vi "Configuration.vi"(11 "Configuration Queue":refnum<queue>) -> ()   [LabVIEW 2013, in "main.lvlib"]
uses:
  main.lvlib
  Controls/Reference AE Control.ctl
  Controls/Reference Cluster.ctl
panel:
  in  "ActivityBox":bool caption="Arbejdstest"
  out "SegmentNumberString":string caption="Nummer"
  out "UndersøgelsesString":string caption="Undersøgelse"
  out "ArmtrykString":string caption="Armtryk"
  in  "Stop":bool
  in  "ListboxLeftSegmentNr":i32(listbox) caption="Venstre"
  in  "ListboxRightSegmentNr":i32(listbox) caption="Højre"
  in  "ListboxMeasurementArea":i32(listbox) caption="Segment"
  in  "ListboxMeasurementTechnique":i32(listbox) caption="Teknik"
  in  "ListboxMeasurementMeth":i32(listbox) caption="Metode"
  in  "TempTwo":dbl caption="#2"
  in  "TempOne":dbl caption="Temperatur"
  in  "PalpationLeft":string(combo)="None" caption="Palpation"
  in  "PalpationRight":string(combo)="None" caption="Palpation"
  in  "LeftArmPressureTable":string[][](table) caption="Venstre"
  in  "RightArmPressureTable":string[][](table) caption="Højre"
  in  "HeightAdjustmentInt":dbl caption="Højdejustering"
  in  "SaveArmPressureBtn":bool caption="Gem"
  in  "Puls":dbl
  # "#1"
  # "#2"
  # "cm"
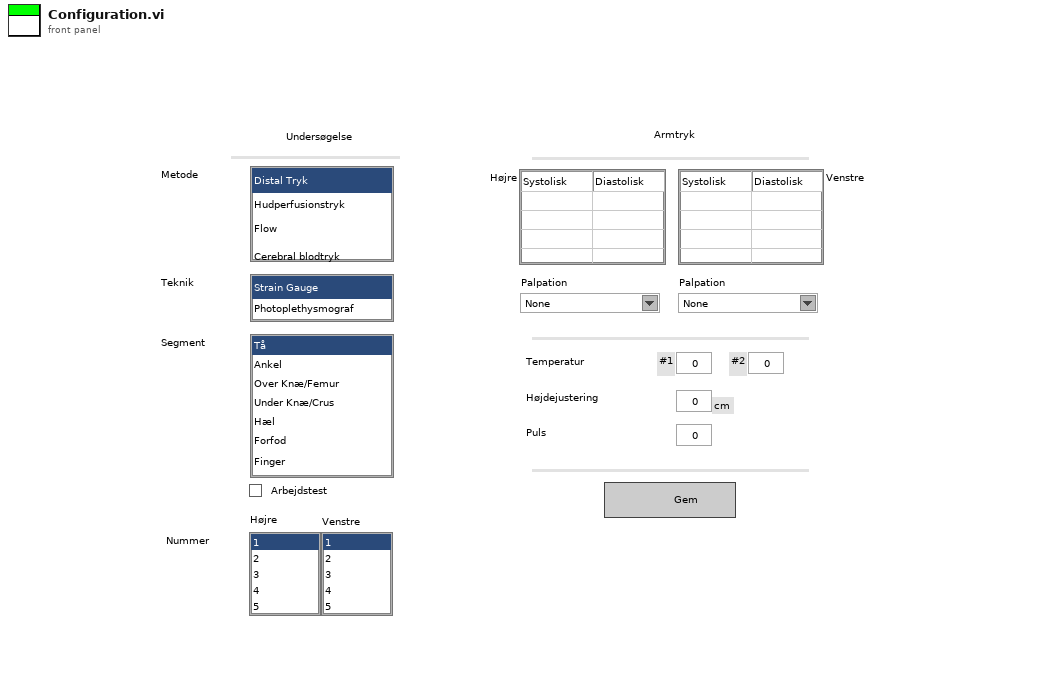
[diagram p1: front panel]
types:
  T1 = typedef "main.lvlib/Reference AE Control.ctl" = enum16{"Initialize", "Set Menu", "Set Profile", "Set Configuration", "Set Configuration_old", "Set Configuration_new", "Set Configuration Method", "Set Acquisition", "Set Data", "Set Journal", "Get"}
  T2 = typedef "main.lvlib/Reference Cluster.ctl" = cluster{"Menu":cluster{"References":cluster{"Stop Acq":refnum<vi>, "MenuExit":refnum<vi>, "MenuStartADC":refnum<vi>, "PersonalInfoString":refnum<vi>, "Profile":refnum<vi>, "Configuration":refnum<vi>, "Acquisition":refnum<vi>, "Data":refnum<vi>, "Journal":refnum<vi>}}, "Profile":cluster{"References":cluster{"Search Patient ID":refnum<vi>, "Name":refnum<vi>, "CommentStr":refnum<vi>, "Listbox Patient ID":refnum<vi>, "ListboxDoctor":refnum<vi>, "ListboxOperator":refnum<vi>, "HospitalName":refnum<vi>, "HospitalDepartment":refnum<vi>, "HospitalAddress":refnum<vi>, "EditHospInfo":refnum<vi>, "Add Patient ID Btn":refnum<vi>, "Query Worklist":refnum<vi>}}, "Configuration":cluster{"References":cluster{"ListboxMeasurementArea":refnum<vi>, "ListboxMeasurementTechnique":refnum<vi>, "ListboxMeasurementMeth":refnum<vi>, "ListboxRightSegmentNr":refnum<vi>, "ListboxLeftSegmentNr":refnum<vi>, "HeightAdjustmentInt":refnum<vi>, "PalpationRight":refnum<vi>, "PalpationLeft":refnum<vi>, "ActivityBox":refnum<vi>}, "New method":cluster{"AddNewMeasurementBtn":refnum<vi>, "Left Time Table":refnum<vi>, "Right Time Table":refnum<vi>}, "Old method":cluster{"LeftArmPressureTable":refnum<vi>, "RightArmPressureTable":refnum<vi>, "SaveArmPressureBtn":refnum<vi>, "Puls":refnum<vi>, "TempTwo":refnum<vi>, "TempOne":refnum<vi>}, "Method":string}, "Acquisition":cluster{"References":cluster{"SegmentAcqString":refnum<vi>, "RingActGraph":refnum<vi>}}, "Data":cluster{"References":cluster{"cmString":refnum<vi>, "AdjustedHeight":refnum<vi>, "Menu":refnum<vi>, "Tangent On/Off":refnum<vi>, "FilterControl":refnum<vi>}}, "Journal":cluster{"References":cluster{"ReportSelection":refnum<vi>, "Data":refnum<vi>, "GenerateReport":refnum<vi>, "Menu":refnum<vi>, "Send To PACS":refnum<vi>}}}
  T3 = cluster{"ListboxMeasurementArea":refnum<vi>, "ListboxMeasurementTechnique":refnum<vi>, "ListboxMeasurementMeth":refnum<vi>, "ListboxRightSegmentNr":refnum<vi>, "ListboxLeftSegmentNr":refnum<vi>, "HeightAdjustmentInt":refnum<vi>, "PalpationRight":refnum<vi>, "PalpationLeft":refnum<vi>, "ActivityBox":refnum<vi>}
  T4 = typedef "LVRectTypeDef.ctl" = cluster{"Left":i16, "Top":i16, "Right":i16, "Bottom":i16}
  T5 = cluster{"sys":dbl, "dia":dbl, "puls":dbl, "date":string, "time":string, "code":string, "serial":string, "temp":dbl, "activity":string}[]
  T6 = cluster{"LeftArmPressureTable":refnum<vi>, "RightArmPressureTable":refnum<vi>, "SaveArmPressureBtn":refnum<vi>, "Puls":refnum<vi>, "TempTwo":refnum<vi>, "TempOne":refnum<vi>}
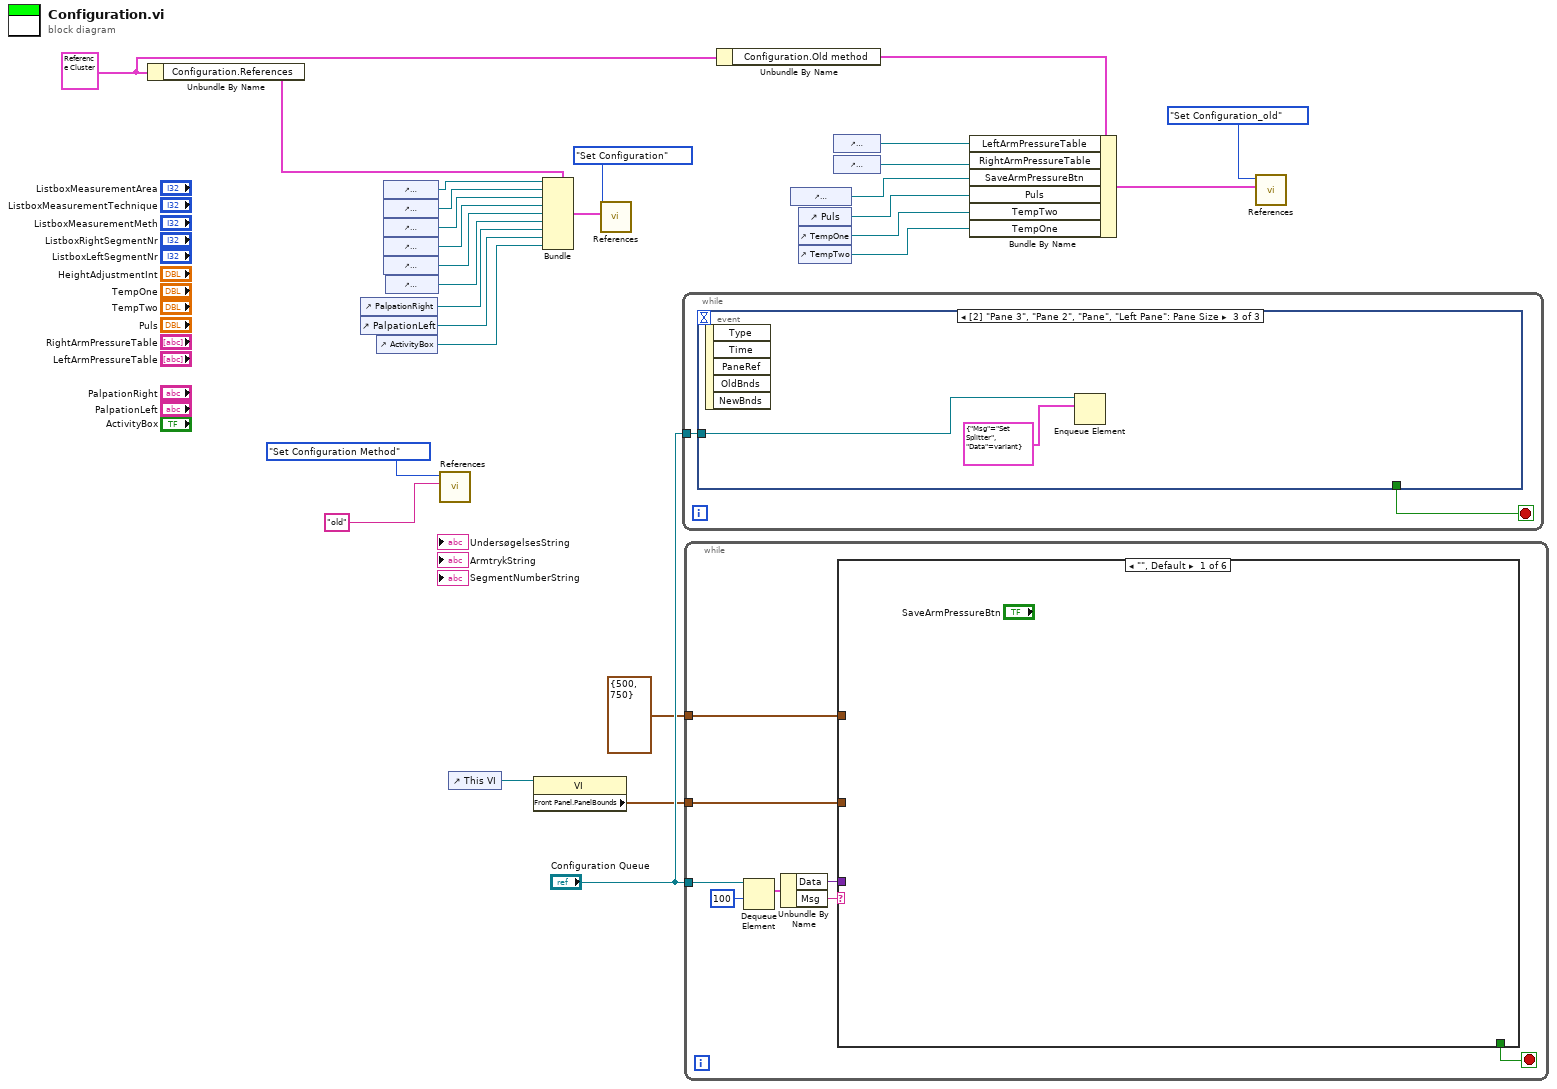
[diagram p0: block diagram]
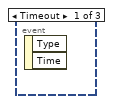
[diagram p2: hidden frame]
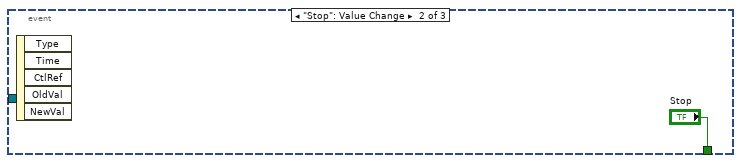
[diagram p3: hidden frame]
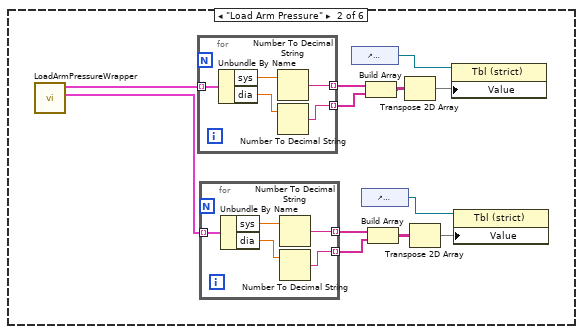
[diagram p4: hidden frame]
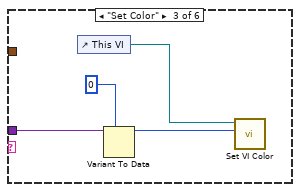
[diagram p5: hidden frame]
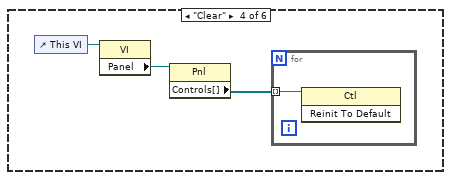
[diagram p6: hidden frame]
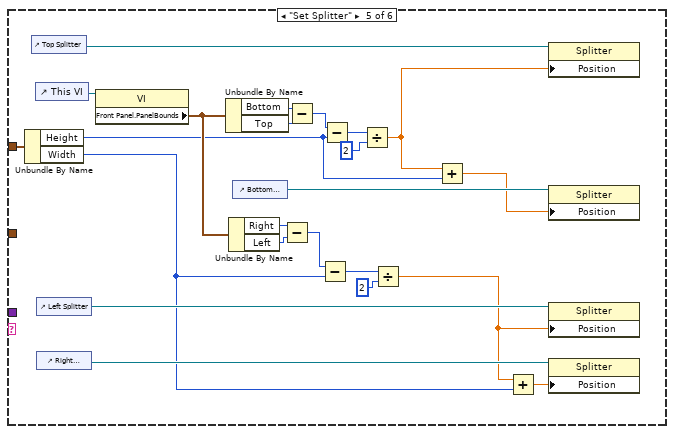
[diagram p7: hidden frame]
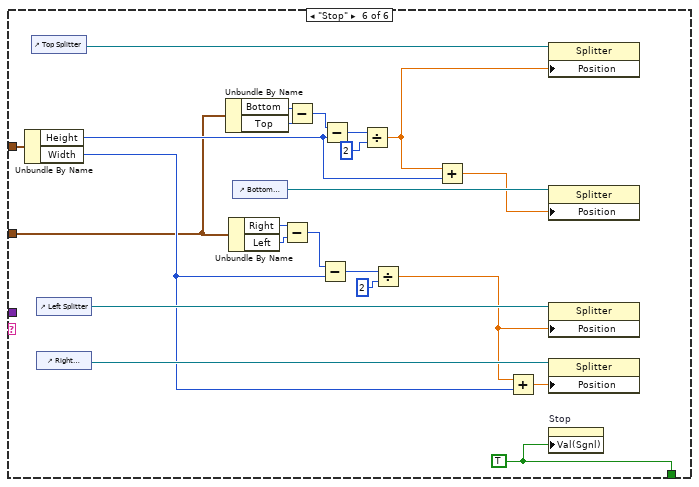
[diagram p8: hidden frame]
diagram:
  w15 = T2 {"Menu"={"References"={"Stop Acq"=refnum, "MenuExit"=refnum, "MenuStartADC"=refnum, "PersonalInfoString"=refnum, "Profile"=refnum, "Configuration"=refnum, "Acquisition"=refnum, "Data"=refnum, "Journal"=refnum}}, "Profile"={"References"={"Search Patient ID"=refnum, "Name"=refnum, "CommentStr"=refnum, "Listbox Patient ID"=refnum, "ListboxDoctor"=refnum, "ListboxOperator"=refnum, "HospitalName"=refnum, "HospitalDepartment"=refnum, "HospitalAddress"=refnum, "EditHospInfo"=refnum, "Add Patient ID Btn"=refnum, "Query Worklist"=refnum}}, "Configuration"={"References"={"ListboxMeasurementArea"=refnum, "ListboxMeasurementTechnique"=refnum, "ListboxMeasurementMeth"=refnum, "ListboxRightSegmentNr"=refnum, "ListboxLeftSegmentNr"=refnum, "HeightAdjustmentInt"=refnum, "PalpationRight"=refnum, "PalpationLeft"=refnum, "ActivityBox"=refnum}, "New method"={"AddNewMeasurementBtn"=refnum, "Left Time Table"=refnum, "Right Time Table"=refnum}, "Old method"={"LeftArmPressureTable"=refnum, "RightArmPressureTable"=refnum, "SaveArmPressureBtn"=refnum, "Puls"=refnum, "TempTwo"=refnum, "TempOne"=refnum}, "Method"=""}, "Acquisition"={"References"={"SegmentAcqString"=refnum, "RingActGraph"=refnum}}, "Data"={"References"={"cmString"=refnum, "AdjustedHeight"=refnum, "Menu"=refnum, "Tangent On/Off"=refnum, "FilterControl"=refnum}}, "Journal"={"References"={"ReportSelection"=refnum, "Data"=refnum, "GenerateReport"=refnum, "Menu"=refnum, "Send To PACS"=refnum}}}
  n1 = Unbundle By Name(w15) -> ("Configuration.References"=w16:T3)
  n2 = control-ref of="PalpationRight"() -> (w5:refnum<vi>)
  n3 = control-ref of="PalpationLeft"() -> (w4:refnum<vi>)
  n4 = control-ref of="ActivityBox"() -> (w3:refnum<vi>)
  n5 = control-ref of="ListboxMeasurementArea"() -> (w28:refnum<vi>)
  n6 = control-ref of="ListboxMeasurementTechnique"() -> (w27:refnum<vi>)
  n7 = control-ref of="ListboxMeasurementMeth"() -> (w26:refnum<vi>)
  n8 = control-ref of="ListboxRightSegmentNr"() -> (w25:refnum<vi>)
  n9 = control-ref of="ListboxLeftSegmentNr"() -> (w24:refnum<vi>)
  n10 = control-ref of="HeightAdjustmentInt"() -> (w23:refnum<vi>)
  n11 = call "References.vi"("variant"="old", "Reference AE Control"=Reference_AE_Control."Set Configuration Method") -> ()  [unwired: 8 in, 2 out]
  n12 = control-ref of="This VI"() -> (w19:refnum<vi>)
  n13 = property class="VI"(reference=w19) -> ("Front Panel.PanelBounds"=w18:T4)  [unwired: 1 in, 2 out]
  n14 = Bundle(cluster=w16, "ListboxMeasurementArea"=w28, "ListboxMeasurementTechnique"=w27, "ListboxMeasurementMeth"=w26, "ListboxRightSegmentNr"=w25, "ListboxLeftSegmentNr"=w24, "HeightAdjustmentInt"=w23, "PalpationRight"=w5, "PalpationLeft"=w4, "ActivityBox"=w3) -> (w21:T3)
  n15 = call "References.vi"("variant"=w21, "Reference AE Control"=Reference_AE_Control."Set Configuration") -> ()  [unwired: 8 in, 2 out]
  n16 = while {
    tunnel: "Configuration Queue" -> [w30]
    stop <- w29 stop-if-true
    n17 = event shown="[2] \"Pane 3\", \"Pane 2\", \"Pane\", \"Left Pane\": Pane Size" {
      selector: _ -> [_ _ _]
      dyn-events: _ -> [_ _ _]
      timeout: _ -> [_ _ _]
      tunnel: w30 -> [_ _ w33]
      tunnel: [_ "Stop" _] -> w29
      event Timeout {
        n18 = event-data() -> ()  [unwired: 1 in, 2 out]
      }
      event "Stop": Value Change {
        n19 = event-data() -> ()  [unwired: 1 in, 5 out]
      }
      event Pane Size {
        n20 = event-data() -> ()  [unwired: 1 in, 5 out]
        n21 = Enqueue Element(queue=w33, element=cluster{"Msg":string, "Data":variant} {"Msg"="Set Splitter", "Data"=variant}) -> ()  [unwired: 2 in, 3 out]
      }
    }
  }
  n22 = while {
    tunnel: "Configuration Queue" -> [w41]
    tunnel: cluster{"Height":i32, "Width":i32} {"Height"=500, "Width"=750} -> [w35]
    tunnel: w18 -> [w34]
    stop <- w38 stop-if-true
    n23 = Dequeue Element(queue=w41, timeout in ms (-1)=100) -> (element=w40:cluster{"Msg":string, "Data":variant})  [unwired: 1 in, 3 out]
    n24 = Unbundle By Name(w40) -> ("Data"=w37:variant, "Msg"=w39:string)
    n25 = case shown="\"\", Default" w39 {
      tunnel: [_ _ _ _ _ w96] -> w38
      tunnel: w37 -> [_ _ w64 _ _ _]
      tunnel: w35 -> [_ _ _ _ w80 w105]
      tunnel: w34 -> [_ _ _ _ _ w95]
      frame "", Default {
      }
      frame "Load Arm Pressure" {
        n26 = call "LoadArmPressureWrapper.vi"() -> ("Armpressure Left"=w48:T5, "Armpressure Right"=w53:T5)  [unwired: 9 in, 1 out]
        n27 = for {
          tunnel: w53 -> [w63] mode=indexing
          tunnel: [w60] -> w52 mode=indexing
          tunnel: [w59] -> w51 mode=indexing
          n28 = Unbundle By Name(w63) -> ("sys"=w62:dbl, "dia"=w61:dbl)
          n29 = Number To Decimal String(number=w62) -> (decimal integer string=w60:string)  [unwired: 1 in]
          n30 = Number To Decimal String(number=w61) -> (decimal integer string=w59:string)  [unwired: 1 in]
        }
        n31 = for {
          tunnel: w48 -> [w58] mode=indexing
          tunnel: [w55] -> w49 mode=indexing
          tunnel: [w54] -> w47 mode=indexing
          n32 = Unbundle By Name(w58) -> ("sys"=w57:dbl, "dia"=w56:dbl)
          n33 = Number To Decimal String(number=w57) -> (decimal integer string=w55:string)  [unwired: 1 in]
          n34 = Number To Decimal String(number=w56) -> (decimal integer string=w54:string)  [unwired: 1 in]
        }
        n35 = control-ref of="RightArmPressureTable"() -> (w50:refnum<vi>)
        n36 = control-ref of="LeftArmPressureTable"() -> (w46:refnum<vi>)
        n37 = Build Array(w52, w51) -> (w45:string[][])
        n38 = Build Array(w49, w47) -> (w43:string[][])
        n39 = Transpose 2D Array(2D array=w45) -> (transposed array=w44:string[][])
        n40 = Transpose 2D Array(2D array=w43) -> (transposed array=w42:string[][])
        n41 = property class="Tbl (strict)"(reference=w50, "Value"=w44) -> ()  [unwired: 1 in, 2 out]
        n42 = property class="Tbl (strict)"(reference=w46, "Value"=w42) -> ()  [unwired: 1 in, 2 out]
      }
      frame "Set Color" {
        n43 = control-ref of="This VI"() -> (w67:refnum<vi>)
        n44 = Variant To Data(type=u32 0 ("Pane Color"), Variant=w64) -> (data=w65:u32)  [unwired: 1 in, 1 out]
        n45 = call "Set VI Color.vi"("Pane Color"=w65, "VI in"=w67) -> ()  [unwired: 10 in]
      }
      frame "Clear" {
        n46 = control-ref of="This VI"() -> (w70:refnum<vi>)
        n47 = property class="VI"(reference=w70) -> ("Panel"=w69:refnum<vi>)  [unwired: 1 in, 2 out]
        n48 = property class="Pnl"(reference=w69) -> ("Controls[]"=w68:refnum<vi>[])  [unwired: 1 in, 2 out]
        n49 = for {
          tunnel: w68 -> [w71] mode=indexing
          n50 = invoke class="Ctl" method="Reinit To Default"(reference=w71) -> ()  [unwired: 2 in, 3 out]
        }
      }
      frame "Set Splitter" {
        n51 = Unbundle By Name(w80) -> ("Height"=w78:i32, "Width"=w73:i32)
        n52 = control-ref of="Top Splitter"() -> (w88:refnum<vi>)
        n53 = control-ref of="This VI"() -> (w94:refnum<vi>)
        n54 = control-ref of="Left Splitter"() -> (w81:refnum<vi>)
        n55 = control-ref of="Right Splitter"() -> (w75:refnum<vi>)
        n56 = property class="VI"(reference=w94) -> ("Front Panel.PanelBounds"=w87:T4)  [unwired: 1 in, 2 out]
        n57 = Unbundle By Name(w87) -> ("Bottom"=w93:i16, "Top"=w92:i16)
        n58 = Unbundle By Name(w87) -> ("Right"=w86:i16, "Left"=w85:i16)
        n59 = control-ref of="Bottom Splitter"() -> (w77:refnum<vi>)
        n60 = Subtract(x=w86, y=w85) -> (x-y=w84:i16)
        n61 = Subtract(x=w93, y=w92) -> (x-y=w91:i16)
        n62 = Subtract(x=w84, y=w73) -> (x-y=w83:i32)
        n63 = Subtract(x=w91, y=w78) -> (x-y=w90:i32)
        n64 = Divide(x=w90, y=2) -> (x/y=w79:dbl)
        n65 = Divide(x=w83, y=u32 2) -> (x/y=w74:dbl)
        n66 = Add(x=w79, y=w78) -> (x+y=w76:dbl)
        n67 = Add(x=w74, y=w73) -> (x+y=w72:dbl)
        n68 = property class="Splitter"(reference=w88, "Position"=w79) -> ()  [unwired: 1 in, 2 out]
        n69 = property class="Splitter"(reference=w77, "Position"=w76) -> ()  [unwired: 1 in, 2 out]
        n70 = property class="Splitter"(reference=w81, "Position"=w74) -> ()  [unwired: 1 in, 2 out]
        n71 = property class="Splitter"(reference=w75, "Position"=w72) -> ()  [unwired: 1 in, 2 out]
      }
      frame "Stop" {
        w96 = TRUE
        n72 = Unbundle By Name(w105) -> ("Height"=w103:i32, "Width"=w98:i32)
        n73 = control-ref of="Top Splitter"() -> (w112:refnum<vi>)
        n74 = control-ref of="Left Splitter"() -> (w106:refnum<vi>)
        n75 = control-ref of="Right Splitter"() -> (w100:refnum<vi>)
        n76 = Unbundle By Name(w95) -> ("Bottom"=w117:i16, "Top"=w116:i16)
        n77 = Unbundle By Name(w95) -> ("Right"=w111:i16, "Left"=w110:i16)
        n78 = control-ref of="Bottom Splitter"() -> (w102:refnum<vi>)
        n79 = Subtract(x=w111, y=w110) -> (x-y=w109:i16)
        n80 = Subtract(x=w117, y=w116) -> (x-y=w115:i16)
        n81 = Subtract(x=w109, y=w98) -> (x-y=w108:i32)
        n82 = Subtract(x=w115, y=w103) -> (x-y=w114:i32)
        n83 = Divide(x=w114, y=2) -> (x/y=w104:dbl)
        n84 = Divide(x=w108, y=u32 2) -> (x/y=w99:dbl)
        n85 = Add(x=w104, y=w103) -> (x+y=w101:dbl)
        n86 = Add(x=w99, y=w98) -> (x+y=w97:dbl)
        n87 = property class="Splitter"(reference=w112, "Position"=w104) -> ()  [unwired: 1 in, 2 out]
        n88 = property class="Splitter"(reference=w102, "Position"=w101) -> ()  [unwired: 1 in, 2 out]
        n89 = property class="Splitter"(reference=w106, "Position"=w99) -> ()  [unwired: 1 in, 2 out]
        n90 = property class="Splitter"(reference=w100, "Position"=w97) -> ()  [unwired: 1 in, 2 out]
        n91 = property on="Stop" class="Bool (strict)"("Val(Sgnl)"=w96) -> ()  [unwired: 2 in, 2 out]
      }
    }
  }
  n92 = Unbundle By Name(w15) -> ("Configuration.Old method"=w14:T6)
  n93 = control-ref of="SaveArmPressureBtn"() -> (w6:refnum<vi>)
  n94 = control-ref of="Puls"() -> (w7:refnum<vi>)
  n95 = control-ref of="TempOne"() -> (w11:refnum<vi>)
  n96 = control-ref of="TempTwo"() -> (w10:refnum<vi>)
  n97 = control-ref of="LeftArmPressureTable"() -> (w9:refnum<vi>)
  n98 = control-ref of="RightArmPressureTable"() -> (w8:refnum<vi>)
  n99 = Bundle By Name(cluster=w14, "LeftArmPressureTable"=w9, "RightArmPressureTable"=w8, "SaveArmPressureBtn"=w6, "Puls"=w7, "TempTwo"=w11, "TempOne"=w10) -> (w13:T6)
  n100 = call "References.vi"("variant"=w13, "Reference AE Control"=Reference_AE_Control."Set Configuration_old") -> ()  [unwired: 8 in, 2 out]
